vi "Test - Draw Teapot.vi"() -> ()   [LabVIEW 2022 SP3, in "Raster.lvlib"] (continued)
"y"=282.48926, "z"=0.9893855}, "UV"={"u"=0.0, "v"=0.0}, "Colour"=12517256}, "Vertex 2"={"Position"={"x"=187.54259, "y"=266.03958, "z"=0.9893693}, "UV"={"u"=0.0, "v"=0.0}, "Colour"=12517256}, "Vertex 3"={"Position"={"x"=198.46721, "y"=268.20078, "z"=0.990049}, "UV"={"u"=0.0, "v"=0.0}, "Colour"=12517256}, "Alpha"=0.0, "Alpha Blending Enabled"=FALSE, "Colour"=3162146}, {"Vertex 1"={"Position"={"x"=612.4574, "y"=266.03958, "z"=0.9893693}, "UV"={"u"=0.0, "v"=0.0}, "Colour"=12517256}, "Vertex 2"={"Position"={"x"=607.4049, "y"=282.48926, "z"=0.9893855}, "UV"={"u"=0.0, "v"=0.0}, "Colour"=12517256}, "Vertex 3"={"Position"={"x"=597.03815, "y"=283.57877, "z"=0.990049}, "UV"={"u"=0.0, "v"=0.0}, "Colour"=12517256}, "Alpha"=0.0, "Alpha Blending Enabled"=FALSE, "Colour"=3162146}, {"Vertex 1"={"Position"={"x"=430.5626, "y"=409.63797, "z"=0.98946077}, "UV"={"u"=0.0, "v"=0.0}, "Colour"=12517256}, "Vertex 2"={"Position"={"x"=421.46735, "y"=411.46152, "z"=0.9896358}, "UV"={"u"=0.0, "v"=0.0}, "Colour"=12517256}, "Vertex 3"={"Position"={"x"=424.30502, "y"=410.7137, "z"=0.9897057}, "UV"={"u"=0.0, "v"=0.0}, "Colour"=12517256}, "Alpha"=0.0, "Alpha Blending Enabled"=FALSE, "Colour"=10145390}, {"Vertex 1"={"Position"={"x"=385.91513, "y"=432.98935, "z"=0.9896798}, "UV"={"u"=0.0, "v"=0.0}, "Colour"=12517256}, "Vertex 2"={"Position"={"x"=382.30276, "y"=440.7109, "z"=0.9895852}, "UV"={"u"=0.0, "v"=0.0}, "Colour"=12517256}, "Vertex 3"={"Position"={"x"=386.13464, "y"=441.3613, "z"=0.9895369}, "UV"={"u"=0.0, "v"=0.0}, "Colour"=12517256}, "Alpha"=0.0, "Alpha Blending Enabled"=FALSE, "Colour"=131841}, {"Vertex 1"={"Position"={"x"=186.5184, "y"=191.99817, "z"=0.98936605}, "UV"={"u"=0.0, "v"=0.0}, "Colour"=12517256}, "Vertex 2"={"Position"={"x"=193.06175, "y"=180.83313, "z"=0.989387}, "UV"={"u"=0.0, "v"=0.0}, "Colour"=12517256}, "Vertex 3"={"Position"={"x"=203.37758, "y"=188.23193, "z"=0.990049}, "UV"={"u"=0.0, "v"=0.0}, "Colour"=12517256}, "Alpha"=0.0, "Alpha Blending Enabled"=FALSE, "Colour"=131841}, {"Vertex 1"={"Position"={"x"=606.9383, "y"=180.83313, "z"=0.989387}, "UV"={"u"=0.0, "v"=0.0}, "Colour"=12517256}, "Vertex 2"={"Position"={"x"=613.4816, "y"=191.99817, "z"=0.98936605}, "UV"={"u"=0.0, "v"=0.0}, "Colour"=12517256}, "Vertex 3"={"Position"={"x"=602.44214, "y"=198.90225, "z"=0.990049}, "UV"={"u"=0.0, "v"=0.0}, "Colour"=12517256}, "Alpha"=0.0, "Alpha Blending Enabled"=FALSE, "Colour"=131841}, {"Vertex 1"={"Position"={"x"=425.17258, "y"=447.3146, "z"=0.98956454}, "UV"={"u"=0.0, "v"=0.0}, "Colour"=12517256}, "Vertex 2"={"Position"={"x"=421.02798, "y"=439.917, "z"=0.9896443}, "UV"={"u"=0.0, "v"=0.0}, "Colour"=12517256}, "Vertex 3"={"Position"={"x"=417.69724, "y"=440.7109, "z"=0.9895852}, "UV"={"u"=0.0, "v"=0.0}, "Colour"=12517256}, "Alpha"=0.0, "Alpha Blending Enabled"=FALSE, "Colour"=131841}, {"Vertex 1"={"Position"={"x"=299.91116, "y"=121.74838, "z"=0.98940194}, "UV"={"u"=0.0, "v"=0.0}, "Colour"=12517256}, "Vertex 2"={"Position"={"x"=327.3322, "y"=123.64719, "z"=0.9895792}, "UV"={"u"=0.0, "v"=0.0}, "Colour"=12517256}, "Vertex 3"={"Position"={"x"=326.15854, "y"=127.58133, "z"=0.9898128}, "UV"={"u"=0.0, "v"=0.0}, "Colour"=12517256}, "Alpha"=0.0, "Alpha Blending Enabled"=FALSE, "Colour"=131841}, {"Vertex 1"={"Position"={"x"=413.86533, "y"=441.3613, "z"=0.9895369}, "UV"={"u"=0.0, "v"=0.0}, "Colour"=12517256}, "Vertex 2"={"Position"={"x"=411.0237, "y"=433.47845, "z"=0.9896417}, "UV"={"u"=0.0, "v"=0.0}, "Colour"=12517256}, "Vertex 3"={"Position"={"x"=407.6209, "y"=433.84442, "z"=0.9896132}, "UV"={"u"=0.0, "v"=0.0}, "Colour"=12517256}, "Alpha"=0.0, "Alpha Blending Enabled"=FALSE, "Colour"=131842}, {"Vertex 1"={"Position"={"x"=521.88995, "y"=127.45417, "z"=0.9896591}, "UV"={"u"=0.0, "v"=0.0}, "Colour"=12517256}, "Vertex 2"={"Position"={"x"=500.85635, "y"=127.179695, "z"=0.98972636}, "UV"={"u"=0.0, "v"=0.0}, "Colour"=12517256}, "Vertex 3"={"Position"={"x"=500.08884, "y"=121.74838, "z"=0.98940194}, "UV"={"u"=0.0, "v"=0.0}, "Colour"=12517256}, "Alpha"=0.0, "Alpha Blending Enabled"=FALSE, "Colour"=131841}, {"Vertex 1"={"Position"={"x"=677.0391, "y"=342.4919, "z"=0.9896034}, "UV"={"u"=0.0, "v"=0.0}, "Colour"=12517256}, "Vertex 2"={"Position"={"x"=673.70026, "y"=326.4925, "z"=0.98952615}, "UV"={"u"=0.0, "v"=0.0}, "Colour"=12517256}, "Vertex 3"={"Position"={"x"=666.5026, "y"=329.28787, "z"=0.9896555}, "UV"={"u"=0.0, "v"=0.0}, "Colour"=12517256}, "Alpha"=0.0, "Alpha Blending Enabled"=FALSE, "Colour"=8696158}, {"Vertex 1"={"Position"={"x"=282.90906, "y"=394.1647, "z"=0.98967445}, "UV"={"u"=0.0, "v"=0.0}, "Colour"=12517256}, "Vertex 2"={"Position"={"x"=297.17767, "y"=396.39102, "z"=0.98972005}, "UV"={"u"=0.0, "v"=0.0}, "Colour"=12517256}, "Vertex 3"={"Position"={"x"=297.89752, "y"=399.48126, "z"=0.9893889}, "UV"={"u"=0.0, "v"=0.0}, "Colour"=12517256}, "Alpha"=0.0, "Alpha Blending Enabled"=FALSE, "Colour"=9091427}, {"Vertex 1"={"Position"={"x"=426.9856, "y"=460.57834, "z"=0.9896675}, "UV"={"u"=0.0, "v"=0.0}, "Colour"=12517256}, "Vertex 2"={"Position"={"x"=431.49448, "y"=457.60767, "z"=0.98960376}, "UV"={"u"=0.0, "v"=0.0}, "Colour"=12517256}, "Vertex 3"={"Position"={"x"=427.8845, "y"=458.98697, "z"=0.9895123}, "UV"={"u"=0.0, "v"=0.0}, "Colour"=12517256}, "Alpha"=0.0, "Alpha Blending Enabled"=FALSE, "Colour"=10540914}, {"Vertex 1"={"Position"={"x"=390.02243, "y"=415.3864, "z"=0.9896799}, "UV"={"u"=0.0, "v"=0.0}, "Colour"=12517256}, "Vertex 2"={"Position"={"x"=385.85406, "y"=412.64026, "z"=0.98952574}, "UV"={"u"=0.0, "v"=0.0}, "Colour"=12517256}, "Vertex 3"={"Position"={"x"=381.9381, "y"=412.10922, "z"=0.98957527}, "UV"={"u"=0.0, "v"=0.0}, "Colour"=12517256}, "Alpha"=0.0, "Alpha Blending Enabled"=FALSE, "Colour"=11331451}, {"Vertex 1"={"Position"={"x"=410.90912, "y"=464.3185, "z"=0.98942566}, "UV"={"u"=0.0, "v"=0.0}, "Colour"=12517256}, "Vertex 2"={"Position"={"x"=406.71997, "y"=463.19003, "z"=0.98966503}, "UV"={"u"=0.0, "v"=0.0}, "Colour"=12517256}, "Vertex 3"={"Position"={"x"=409.72174, "y"=462.79736, "z"=0.98969}, "UV"={"u"=0.0, "v"=0.0}, "Colour"=12517256}, "Alpha"=0.0, "Alpha Blending Enabled"=FALSE, "Colour"=10343280}, {"Vertex 1"={"Position"={"x"=390.2171, "y"=413.03857, "z"=0.9894885}, "UV"={"u"=0.0, "v"=0.0}, "Colour"=12517256}, "Vertex 2"={"Position"={"x"=393.107, "y"=415.6739, "z"=0.98965406}, "UV"={"u"=0.0, "v"=0.0}, "Colour"=12517256}, "Vertex 3"={"Position"={"x"=396.44946, "y"=415.85388, "z"=0.98963785}, "UV"={"u"=0.0, "v"=0.0}, "Colour"=12517256}, "Alpha"=0.0, "Alpha Blending Enabled"=FALSE, "Colour"=11792768}, {"Vertex 1"={"Position"={"x"=648.53705, "y"=216.88268, "z"=0.98970413}, "UV"={"u"=0.0, "v"=0.0}, "Colour"=12517256}, "Vertex 2"={"Position"={"x"=621.5498, "y"=201.64421, "z"=0.9896861}, "UV"={"u"=0.0, "v"=0.0}, "Colour"=12517256}, "Vertex 3"={"Position"={"x"=626.93384, "y"=205.09799, "z"=0.989385}, "UV"={"u"=0.0, "v"=0.0}, "Colour"=12517256}, "Alpha"=0.0, "Alpha Blending Enabled"=FALSE, "Colour"=131841}, {"Vertex 1"={"Position"={"x"=187.54259, "y"=266.03958, "z"=0.9893693}, "UV"={"u"=0.0, "v"=0.0}, "Colour"=12517256}, "Vertex 2"={"Position"={"x"=183.7062, "y"=249.90852, "z"=0.98935705}, "UV"={"u"=0.0, "v"=0.0}, "Colour"=12517256}, "Vertex 3"={"Position"={"x"=195.06374, "y"=253.1501, "z"=0.990049}, "UV"={"u"=0.0, "v"=0.0}, "Colour"=12517256}, "Alpha"=0.0, "Alpha Blending Enabled"=FALSE, "Colour"=2635036}, {"Vertex 1"={"Position"={"x"=616.2938, "y"=249.90852, "z"=0.98935705}, "UV"={"u"=0.0, "v"=0.0}, "Colour"=12517256}, "Vertex 2"={"Position"={"x"=612.4574, "y"=266.03958, "z"=0.9893693}, "UV"={"u"=0.0, "v"=0.0}, "Colour"=12517256}, "Vertex 3"={"Position"={"x"=601.5328, "y"=268.20078, "z"=0.990049}, "UV"={"u"=0.0, "v"=0.0}, "Colour"=12517256}, "Alpha"=0.0, "Alpha Blending Enabled"=FALSE, "Colour"=2635036}, {"Vertex 1"={"Position"={"x"=662.8395, "y"=314.53314, "z"=0.9895922}, "UV"={"u"=0.0, "v"=0.0}, "Colour"=12517256}, "Vertex 2"={"Position"={"x"=666.5026, "y"=329.28787, "z"=0.9896555}, "UV"={"u"=0.0, "v"=0.0}, "Colour"=12517256}, "Vertex 3"={"Position"={"x"=673.70026, "y"=326.4925, "z"=0.98952615}, "UV"={"u"=0.0, "v"=0.0}, "Colour"=12517256}, "Alpha"=0.0, "Alpha Blending Enabled"=FALSE, "Colour"=8696158}, {"Vertex 1"={"Position"={"x"=189.80782, "y"=199.68152, "z"=0.98959744}, "UV"={"u"=0.0, "v"=0.0}, "Colour"=12517256}, "Vertex 2"={"Position"={"x"=169.41815, "y"=209.785, "z"=0.98959744}, "UV"={"u"=0.0, "v"=0.0}, "Colour"=12517256}, "Vertex 3"={"Position"={"x"=168.53177, "y"=213.96883, "z"=0.9895778}, "UV"={"u"=0.0, "v"=0.0}, "Colour"=12517256}, "Alpha"=0.0, "Alpha Blending Enabled"=FALSE, "Colour"=6522183}, {"Vertex 1"={"Position"={"x"=168.51642, "y"=218.47636, "z"=0.98959744}, "UV"={"u"=0.0, "v"=0.0}, "Colour"=12517256}, "Vertex 2"={"Position"={"x"=186.59279, "y"=209.32652, "z"=0.98959744}, "UV"={"u"=0.0, "v"=0.0}, "Colour"=12517256}, "Vertex 3"={"Position"={"x"=187.80107, "y"=204.32404, "z"=0.9895778}, "UV"={"u"=0.0, "v"=0.0}, "Colour"=12517256}, "Alpha"=0.0, "Alpha Blending Enabled"=FALSE, "Colour"=10606707}, {"Vertex 1"={"Position"={"x"=169.41815, "y"=209.785, "z"=0.98959744}, "UV"={"u"=0.0, "v"=0.0}, "Colour"=12517256}, "Vertex 2"={"Position"={"x"=151.36185, "y"=220.60233, "z"=0.98959744}, "UV"={"u"=0.0, "v"=0.0}, "Colour"=12517256}, "Vertex 3"={"Position"={"x"=151.49875, "y"=224.43393, "z"=0.9895778}, "UV"={"u"=0.0, "v"=0.0}, "Colour"=12517256}, "Alpha"=0.0, "Alpha Blending Enabled"=FALSE, "Colour"=6653768}, {"Vertex 1"={"Position"={"x"=152.57072, "y"=228.54994, "z"=0.98959744}, "UV"={"u"=0.0, "v"=0.0}, "Colour"=12517256}, "Vertex 2"={"Position"={"x"=168.51642, "y"=218.47636, "z"=0.98959744}, "UV"={"u"=0.0, "v"=0.0}, "Colour"=12517256}, "Vertex 3"={"Position"={"x"=168.53177, "y"=213.96883, "z"=0.9895778}, "UV"={"u"=0.0, "v"=0.0}, "Colour"=12517256}, "Alpha"=0.0, "Alpha Blending Enabled"=FALSE, "Colour"=10540915}, {"Vertex 1"={"Position"={"x"=151.36185, "y"=220.60233, "z"=0.98959744}, "UV"={"u"=0.0, "v"=0.0}, "Colour"=12517256}, "Vertex 2"={"Position"={"x"=135.59482, "y"=232.01439, "z"=0.98959744}, "UV"={"u"=0.0, "v"=0.0}, "Colour"=12517256}, "Vertex 3"={"Position"={"x"=136.65297, "y"=235.5601, "z"=0.9895778}, "UV"={"u"=0.0, "v"=0.0}, "Colour"=12517256}, "Alpha"=0.0, "Alpha Blending Enabled"=FALSE, "Colour"=6851402}, {"Vertex 1"={"Position"={"x"=138.70209, "y"=239.3482, "z"=0.98959744}, "UV"={"u"=0.0, "v"=0.0}, "Colour"=12517256}, "Vertex 2"={"Position"={"x"=152.57072, "y"=228.54994, "z"=0.98959744}, "UV"={"u"=0.0, "v"=0.0}, "Colour"=12517256}, "Vertex 3"={"Position"={"x"=151.49875, "y"=224.43393, "z"=0.9895778}, "UV"={"u"=0.0, "v"=0.0}, "Colour"=12517256}, "Alpha"=0.0, "Alpha Blending Enabled"=FALSE, "Colour"=10409073}, {"Vertex 1"={"Position"={"x"=135.59482, "y"=232.01439, "z"=0.98959744}, "UV"={"u"=0.0, "v"=0.0}, "Colour"=12517256}, "Vertex 2"={"Position"={"x"=122.07298, "y"=243.90215, "z"=0.98959744}, "UV"={"u"=0.0, "v"=0.0}, "Colour"=12517256}, "Vertex 3"={"Position"={"x"=123.94555, "y"=247.18822, "z"=0.9895778}, "UV"={"u"=0.0, "v"=0.0}, "Colour"=12517256}, "Alpha"=0.0, "Alpha Blending Enabled"=FALSE, "Colour"=7049293}, {"Vertex 1"={"Position"={"x"=126.85683, "y"=250.67299, "z"=0.98959744}, "UV"={"u"=0.0, "v"=0.0}, "Colour"=12517256}, "Vertex 2"={"Position"={"x"=138.70209, "y"=239.3482, "z"=0.98959744}, "UV"={"u"=0.0, "v"=0.0}, "Colour"=12517256}, "Vertex 3"={"Position"={"x"=136.65297, "y"=235.5601, "z"=0.9895778}, "UV"={"u"=0.0, "v"=0.0}, "Colour"=12517256}, "Alpha"=0.0, "Alpha Blending Enabled"=FALSE, "Colour"=10211183}, {"Vertex 1"={"Position"={"x"=122.07298, "y"=243.90215, "z"=0.98959744}, "UV"={"u"=0.0, "v"=0.0}, "Colour"=12517256}, "Vertex 2"={"Position"={"x"=110.75225, "y"=256.14658, "z"=0.98959744}, "UV"={"u"=0.0, "v"=0.0}, "Colour"=12517256}, "Vertex 3"={"Position"={"x"=113.32741, "y"=259.15903, "z"=0.9895778}, "UV"={"u"=0.0, "v"=0.0}, "Colour"=12517256}, "Alpha"=0.0, "Alpha Blending Enabled"=FALSE, "Colour"=7312720}, {"Vertex 1"={"Position"={"x"=116.981316, "y"=262.32532, "z"=0.98959744}, "UV"={"u"=0.0, "v"=0.0}, "Colour"=12517256}, "Vertex 2"={"Position"={"x"=126.85683, "y"=250.67299, "z"=0.98959744}, "UV"={"u"=0.0, "v"=0.0}, "Colour"=12517256}, "Vertex 3"={"Position"={"x"=123.94555, "y"=247.18822, "z"=0.9895778}, "UV"={"u"=0.0, "v"=0.0}, "Colour"=12517256}, "Alpha"=0.0, "Alpha Blending Enabled"=FALSE, "Colour"=9948012}, {"Vertex 1"={"Position"={"x"=110.75225, "y"=256.14658, "z"=0.98959744}, "UV"={"u"=0.0, "v"=0.0}, "Colour"=12517256}, "Vertex 2"={"Position"={"x"=101.588585, "y"=268.6284, "z"=0.98959744}, "UV"={"u"=0.0, "v"=0.0}, "Colour"=12517256}, "Vertex 3"={"Position"={"x"=104.74968, "y"=271.31357, "z"=0.9895778}, "UV"={"u"=0.0, "v"=0.0}, "Colour"=12517256}, "Alpha"=0.0, "Alpha Blending Enabled"=FALSE, "Colour"=7576146}, {"Vertex 1"={"Position"={"x"=109.02176, "y"=274.10672, "z"=0.98959744}, "UV"={"u"=0.0, "v"=0.0}, "Colour"=12517256}, "Vertex 2"={"Position"={"x"=116.981316, "y"=262.32532, "z"=0.98959744}, "UV"={"u"=0.0, "v"=0.0}, "Colour"=12517256}, "Vertex 3"={"Position"={"x"=113.32741, "y"=259.15903, "z"=0.9895778}, "UV"={"u"=0.0, "v"=0.0}, "Colour"=12517256}, "Alpha"=0.0, "Alpha Blending Enabled"=FALSE, "Colour"=9750122}, {"Vertex 1"={"Position"={"x"=101.588585, "y"=268.6284, "z"=0.98959744}, "UV"={"u"=0.0, "v"=0.0}, "Colour"=12517256}, "Vertex 2"={"Position"={"x"=94.53805, "y"=281.22873, "z"=0.98959744}, "UV"={"u"=0.0, "v"=0.0}, "Colour"=12517256}, "Vertex 3"={"Position"={"x"=98.163345, "y"=283.49265, "z"=0.9895778}, "UV"={"u"=0.0, "v"=0.0}, "Colour"=12517256}, "Alpha"=0.0, "Alpha Blending Enabled"=FALSE, "Colour"=7774037}, {"Vertex 1"={"Position"={"x"=102.92444, "y"=285.8186, "z"=0.98959744}, "UV"={"u"=0.0, "v"=0.0}, "Colour"=12517256}, "Vertex 2"={"Position"={"x"=109.02176, "y"=274.10672, "z"=0.98959744}, "UV"={"u"=0.0, "v"=0.0}, "Colour"=12517256}, "Vertex 3"={"Position"={"x"=104.74968, "y"=271.31357, "z"=0.9895778}, "UV"={"u"=0.0, "v"=0.0}, "Colour"=12517256}, "Alpha"=0.0, "Alpha Blending Enabled"=FALSE, "Colour"=9486951}, {"Vertex 1"={"Position"={"x"=94.53805, "y"=281.22873, "z"=0.98959744}, "UV"={"u"=0.0, "v"=0.0}, "Colour"=12517256}, "Vertex 2"={"Position"={"x"=89.5565, "y"=293.82855, "z"=0.98959744}, "UV"={"u"=0.0, "v"=0.0}, "Colour"=12517256}, "Vertex 3"={"Position"={"x"=93.51947, "y"=295.5369, "z"=0.9895778}, "UV"={"u"=0.0, "v"=0.0}, "Colour"=12517256}, "Alpha"=0.0, "Alpha Blending Enabled"=FALSE, "Colour"=8037463}, {"Vertex 1"={"Position"={"x"=98.63565, "y"=297.2621, "z"=0.98959744}, "UV"={"u"=0.0, "v"=0.0}, "Colour"=12517256}, "Vertex 2"={"Position"={"x"=102.92444, "y"=285.8186, "z"=0.98959744}, "UV"={"u"=0.0, "v"=0.0}, "Colour"=12517256}, "Vertex 3"={"Position"={"x"=98.163345, "y"=283.49265, "z"=0.9895778}, "UV"={"u"=0.0, "v"=0.0}, "Colour"=12517256}, "Alpha"=0.0, "Alpha Blending Enabled"=FALSE, "Colour"=9289061}, {"Vertex 1"={"Position"={"x"=89.5565, "y"=293.82855, "z"=0.98959744}, "UV"={"u"=0.0, "v"=0.0}, "Colour"=12517256}, "Vertex 2"={"Position"={"x"=86.5999, "y"=306.30865, "z"=0.98959744}, "UV"={"u"=0.0, "v"=0.0}, "Colour"=12517256}, "Vertex 3"={"Position"={"x"=90.76903, "y"=307.28738, "z"=0.9895778}, "UV"={"u"=0.0, "v"=0.0}, "Colour"=12517256}, "Alpha"=0.0, "Alpha Blending Enabled"=FALSE, "Colour"=8300890}, {"Vertex 1"={"Position"={"x"=96.10178, "y"=308.23883, "z"=0.98959744}, "UV"={"u"=0.0, "v"=0.0}, "Colour"=12517256}, "Vertex 2"={"Position"={"x"=98.63565, "y"=297.2621, "z"=0.98959744}, "UV"={"u"=0.0, "v"=0.0}, "Colour"=12517256}, "Vertex 3"={"Position"={"x"=93.51947, "y"=295.5369, "z"=0.9895778}, "UV"={"u"=0.0, "v"=0.0}, "Colour"=12517256}, "Alpha"=0.0, "Alpha Blending Enabled"=FALSE, "Colour"=9091427}, {"Vertex 1"={"Position"={"x"=86.5999, "y"=306.30865, "z"=0.98959744}, "UV"={"u"=0.0, "v"=0.0}, "Colour"=12517256}, "Vertex 2"={"Position"={"x"=85.62412, "y"=318.55002, "z"=0.98959744}, "UV"={"u"=0.0, "v"=0.0}, "Colour"=12517256}, "Vertex 3"={"Position"={"x"=89.86314, "y"=318.58496, "z"=0.9895778}, "UV"={"u"=0.0, "v"=0.0}, "Colour"=12517256}, "Alpha"=0.0, "Alpha Blending Enabled"=FALSE, "Colour"=8564317}, {"Vertex 1"={"Position"={"x"=95.26916, "y"=318.55002, "z"=0.98959744}, "UV"={"u"=0.0, "v"=0.0}, "Colour"=12517256}, "Vertex 2"={"Position"={"x"=96.10178, "y"=308.23883, "z"=0.98959744}, "UV"={"u"=0.0, "v"=0.0}, "Colour"=12517256}, "Vertex 3"={"Position"={"x"=90.76903, "y"=307.28738, "z"=0.9895778}, "UV"={"u"=0.0, "v"=0.0}, "Colour"=12517256}, "Alpha"=0.0, "Alpha Blending Enabled"=FALSE, "Colour"=8828000}, {"Vertex 1"={"Position"={"x"=85.62412, "y"=318.55002, "z"=0.98959744}, "UV"={"u"=0.0, "v"=0.0}, "Colour"=12517256}, "Vertex 2"={"Position"={"x"=87.13484, "y"=329.46445, "z"=0.98959744}, "UV"={"u"=0.0, "v"=0.0}, "Colour"=12517256}, "Vertex 3"={"Position"={"x"=91.32674, "y"=328.538, "z"=0.9895778}, "UV"={"u"=0.0, "v"=0.0}, "Colour"=12517256}, "Alpha"=0.0, "Alpha Blending Enabled"=FALSE, "Colour"=8894049}, {"Vertex 1"={"Position"={"x"=96.68016, "y"=327.50403, "z"=0.98959744}, "UV"={"u"=0.0, "v"=0.0}, "Colour"=12517256}, "Vertex 2"={"Position"={"x"=95.26916, "y"=318.55002, "z"=0.98959744}, "UV"={"u"=0.0, "v"=0.0}, "Colour"=12517256}, "Vertex 3"={"Position"={"x"=89.86314, "y"=318.58496, "z"=0.9895778}, "UV"={"u"=0.0, "v"=0.0}, "Colour"=12517256}, "Alpha"=0.0, "Alpha Blending Enabled"=FALSE, "Colour"=8366939}, {"Vertex 1"={"Position"={"x"=87.13484, "y"=329.46445, "z"=0.98959744}, "UV"={"u"=0.0, "v"=0.0}, "Colour"=12517256}, "Vertex 2"={"Position"={"x"=91.65158, "y"=338.20395, "z"=0.98959744}, "UV"={"u"=0.0, "v"=0.0}, "Colour"=12517256}, "Vertex 3"={"Position"={"x"=95.695854, "y"=336.50763, "z"=0.9895778}, "UV"={"u"=0.0, "v"=0.0}, "Colour"=12517256}, "Alpha"=0.0, "Alpha Blending Enabled"=FALSE, "Colour"=9486695}, {"Vertex 1"={"Position"={"x"=100.88518, "y"=334.67392, "z"=0.98959744}, "UV"={"u"=0.0, "v"=0.0}, "Colour"=12517256}, "Vertex 2"={"Position"={"x"=96.68016, "y"=327.50403, "z"=0.98959744}, "UV"={"u"=0.0, "v"=0.0}, "Colour"=12517256}, "Vertex 3"={"Position"={"x"=91.32674, "y"=328.538, "z"=0.9895778}, "UV"={"u"=0.0, "v"=0.0}, "Colour"=12517256}, "Alpha"=0.0, "Alpha Blending Enabled"=FALSE, "Colour"=7707988}, {"Vertex 1"={"Position"={"x"=91.65158, "y"=338.20395, "z"=0.98959744}, "UV"={"u"=0.0, "v"=0.0}, "Colour"=12517256}, "Vertex 2"={"Position"={"x"=99.15168, "y"=345.0104, "z"=0.98959744}, "UV"={"u"=0.0, "v"=0.0}, "Colour"=12517256}, "Vertex 3"={"Position"={"x"=102.93782, "y"=342.71442, "z"=0.9895778}, "UV"={"u"=0.0, "v"=0.0}, "Colour"=12517256}, "Alpha"=0.0, "Alpha Blending Enabled"=FALSE, "Colour"=10013805}, {"Vertex 1"={"Position"={"x"=107.84178, "y"=340.25775, "z"=0.98959744}, "UV"={"u"=0.0, "v"=0.0}, "Colour"=12517256}, "Vertex 2"={"Position"={"x"=100.88518, "y"=334.67392, "z"=0.98959744}, "UV"={"u"=0.0, "v"=0.0}, "Colour"=12517256}, "Vertex 3"={"Position"={"x"=95.695854, "y"=336.50763, "z"=0.9895778}, "UV"={"u"=0.0, "v"=0.0}, "Colour"=12517256}, "Alpha"=0.0, "Alpha Blending Enabled"=FALSE, "Colour"=7114829}, {"Vertex 1"={"Position"={"x"=99.15168, "y"=345.0104, "z"=0.98959744}, "UV"={"u"=0.0, "v"=0.0}, "Colour"=12517256}, "Vertex 2"={"Position"={"x"=109.61189, "y"=350.12524, "z"=0.98959744}, "UV"={"u"=0.0, "v"=0.0}, "Colour"=12517256}, "Vertex 3"={"Position"={"x"=113.01999, "y"=347.37875, "z"=0.9895778}, "UV"={"u"=0.0, "v"=0.0}, "Colour"=12517256}, "Alpha"=0.0, "Alpha Blending Enabled"=FALSE, "Colour"=10409073}, {"Vertex 1"={"Position"={"x"=117.50798, "y"=344.45398, "z"=0.98959744}, "UV"={"u"=0.0, "v"=0.0}, "Colour"=12517256}, "Vertex 2"={"Position"={"x"=107.84178, "y"=340.25775, "z"=0.98959744}, "UV"={"u"=0.0, "v"=0.0}, "Colour"=12517256}, "Vertex 3"={"Position"={"x"=102.93782, "y"=342.71442, "z"=0.9895778}, "UV"={"u"=0.0, "v"=0.0}, "Colour"=12517256}, "Alpha"=0.0, "Alpha Blending Enabled"=FALSE, "Colour"=6588232}, {"Vertex 1"={"Position"={"x"=109.61189, "y"=350.12524, "z"=0.98959744}, "UV"={"u"=0.0, "v"=0.0}, "Colour"=12517256}, "Vertex 2"={"Position"={"x"=123.00947, "y"=353.7902, "z"=0.98959744}, "UV"={"u"=0.0, "v"=0.0}, "Colour"=12517256}, "Vertex 3"={"Position"={"x"=125.90974, "y"=350.72086, "z"=0.9895778}, "UV"={"u"=0.0, "v"=0.0}, "Colour"=12517256}, "Alpha"=0.0, "Alpha Blending Enabled"=FALSE, "Colour"=10672500}, {"Vertex 1"={"Position"={"x"=129.84137, "y"=347.46066, "z"=0.98959744}, "UV"={"u"=0.0, "v"=0.0}, "Colour"=12517256}, "Vertex 2"={"Position"={"x"=117.50798, "y"=344.45398, "z"=0.98959744}, "UV"={"u"=0.0, "v"=0.0}, "Colour"=12517256}, "Vertex 3"={"Position"={"x"=113.01999, "y"=347.37875, "z"=0.9895778}, "UV"={"u"=0.0, "v"=0.0}, "Colour"=12517256}, "Alpha"=0.0, "Alpha Blending Enabled"=FALSE, "Colour"=6324549}, {"Vertex 1"={"Position"={"x"=123.00947, "y"=353.7902, "z"=0.98959744}, "UV"={"u"=0.0, "v"=0.0}, "Colour"=12517256}, "Vertex 2"={"Position"={"x"=139.3214, "y"=356.247, "z"=0.98959744}, "UV"={"u"=0.0, "v"=0.0}, "Colour"=12517256}, "Vertex 3"={"Position"={"x"=141.57439, "y"=352.9612, "z"=0.9895778}, "UV"={"u"=0.0, "v"=0.0}, "Colour"=12517256}, "Alpha"=0.0, "Alpha Blending Enabled"=FALSE, "Colour"=10738549}, {"Vertex 1"={"Position"={"x"=144.79973, "y"=349.47617, "z"=0.98959744}, "UV"={"u"=0.0, "v"=0.0}, "Colour"=12517256}, "Vertex 2"={"Position"={"x"=129.84137, "y"=347.46066, "z"=0.98959744}, "UV"={"u"=0.0, "v"=0.0}, "Colour"=12517256}, "Vertex 3"={"Position"={"x"=125.90974, "y"=350.72086, "z"=0.9895778}, "UV"={"u"=0.0, "v"=0.0}, "Colour"=12517256}, "Alpha"=0.0, "Alpha Blending Enabled"=FALSE, "Colour"=6258500}, {"Vertex 1"={"Position"={"x"=139.3214, "y"=356.247, "z"=0.98959744}, "UV"={"u"=0.0, "v"=0.0}, "Colour"=12517256}, "Vertex 2"={"Position"={"x"=158.52467, "y"=357.73706, "z"=0.98959744}, "UV"={"u"=0.0, "v"=0.0}, "Colour"=12517256}, "Vertex 3"={"Position"={"x"=159.98125, "y"=354.3201, "z"=0.9895778}, "UV"={"u"=0.0, "v"=0.0}, "Colour"=12517256}, "Alpha"=0.0, "Alpha Blending Enabled"=FALSE, "Colour"=10804598}, {"Vertex 1"={"Position"={"x"=162.341, "y"=350.69873, "z"=0.98959744}, "UV"={"u"=0.0, "v"=0.0}, "Colour"=12517256}, "Vertex 2"={"Position"={"x"=144.79973, "y"=349.47617, "z"=0.98959744}, "UV"={"u"=0.0, "v"=0.0}, "Colour"=12517256}, "Vertex 3"={"Position"={"x"=141.57439, "y"=352.9612, "z"=0.9895778}, "UV"={"u"=0.0, "v"=0.0}, "Colour"=12517256}, "Alpha"=0.0, "Alpha Blending Enabled"=FALSE, "Colour"=6192707}, {"Vertex 1"={"Position"={"x"=158.52467, "y"=357.73706, "z"=0.98959744}, "UV"={"u"=0.0, "v"=0.0}, "Colour"=12517256}, "Vertex 2"={"Position"={"x"=180.59659, "y"=358.50238, "z"=0.98959744}, "UV"={"u"=0.0, "v"=0.0}, "Colour"=12517256}, "Vertex 3"={"Position"={"x"=181.09776, "y"=355.0179, "z"=0.9895778}, "UV"={"u"=0.0, "v"=0.0}, "Colour"=12517256}, "Alpha"=0.0, "Alpha Blending Enabled"=FALSE, "Colour"=10870134}, {"Vertex 1"={"Position"={"x"=182.42264, "y"=351.32635, "z"=0.98959744}, "UV"={"u"=0.0, "v"=0.0}, "Colour"=12517256}, "Vertex 2"={"Position"={"x"=162.341, "y"=350.69873, "z"=0.98959744}, "UV"={"u"=0.0, "v"=0.0}, "Colour"=12517256}, "Vertex 3"={"Position"={"x"=159.98125, "y"=354.3201, "z"=0.9895778}, "UV"={"u"=0.0, "v"=0.0}, "Colour"=12517256}, "Alpha"=0.0, "Alpha Blending Enabled"=FALSE, "Colour"=6192707}, {"Vertex 1"={"Position"={"x"=180.59659, "y"=358.50238, "z"=0.98959744}, "UV"={"u"=0.0, "v"=0.0}, "Colour"=12517256}, "Vertex 2"={"Position"={"x"=205.5139, "y"=358.7842, "z"=0.98959744}, "UV"={"u"=0.0, "v"=0.0}, "Colour"=12517256}, "Vertex 3"={"Position"={"x"=204.89125, "y"=355.27502, "z"=0.9895778}, "UV"={"u"=0.0, "v"=0.0}, "Colour"=12517256}, "Alpha"=0.0, "Alpha Blending Enabled"=FALSE, "Colour"=10870134}, {"Vertex 1"={"Position"={"x"=205.00276, "y"=351.5577, "z"=0.98959744}, "UV"={"u"=0.0, "v"=0.0}, "Colour"=12517256}, "Vertex 2"={"Position"={"x"=182.42264, "y"=351.32635, "z"=0.98959744}, "UV"={"u"=0.0, "v"=0.0}, "Colour"=12517256}, "Vertex 3"={"Position"={"x"=181.09776, "y"=355.0179, "z"=0.9895778}, "UV"={"u"=0.0, "v"=0.0}, "Colour"=12517256}, "Alpha"=0.0, "Alpha Blending Enabled"=FALSE, "Colour"=6192964}, {"Vertex 1"={"Position"={"x"=205.5139, "y"=358.7842, "z"=0.98959744}, "UV"={"u"=0.0, "v"=0.0}, "Colour"=12517256}, "Vertex 2"={"Position"={"x"=233.2539, "y"=358.82452, "z"=0.98959744}, "UV"={"u"=0.0, "v"=0.0}, "Colour"=12517256}, "Vertex 3"={"Position"={"x"=231.32906, "y"=355.31174, "z"=0.9895778}, "UV"={"u"=0.0, "v"=0.0}, "Colour"=12517256}, "Alpha"=0.0, "Alpha Blending Enabled"=FALSE, "Colour"=10870134}, {"Vertex 1"={"Position"={"x"=230.03891, "y"=351.59073, "z"=0.98959744}, "UV"={"u"=0.0, "v"=0.0}, "Colour"=12517256}, "Vertex 2"={"Position"={"x"=205.00276, "y"=351.5577, "z"=0.98959744}, "UV"={"u"=0.0, "v"=0.0}, "Colour"=12517256}, "Vertex 3"={"Position"={"x"=204.89125, "y"=355.27502, "z"=0.9895778}, "UV"={"u"=0.0, "v"=0.0}, "Colour"=12517256}, "Alpha"=0.0, "Alpha Blending Enabled"=FALSE, "Colour"=6258500}, {"Vertex 1"={"Position"={"x"=348.88834, "y"=405.76608, "z"=0.98953724}, "UV"={"u"=0.0, "v"=0.0}, "Colour"=12517256}, "Vertex 2"={"Position"={"x"=362.46423, "y"=407.4392, "z"=0.98967314}, "UV"={"u"=0.0, "v"=0.0}, "Colour"=12517256}, "Vertex 3"={"Position"={"x"=365.49564, "y"=408.5937, "z"=0.9895617}, "UV"={"u"=0.0, "v"=0.0}, "Colour"=12517256}, "Alpha"=0.0, "Alpha Blending Enabled"=FALSE, "Colour"=9618536}, {"Vertex 1"={"Position"={"x"=427.8845, "y"=458.98697, "z"=0.9895123}, "UV"={"u"=0.0, "v"=0.0}, "Colour"=12517256}, "Vertex 2"={"Position"={"x"=423.8626, "y"=461.78098, "z"=0.98958975}, "UV"={"u"=0.0, "v"=0.0}, "Colour"=12517256}, "Vertex 3"={"Position"={"x"=426.9856, "y"=460.57834, "z"=0.9896675}, "UV"={"u"=0.0, "v"=0.0}, "Colour"=12517256}, "Alpha"=0.0, "Alpha Blending Enabled"=FALSE, "Colour"=10540914}, {"Vertex 1"={"Position"={"x"=182.0637, "y"=204.669, "z"=0.98935175}, "UV"={"u"=0.0, "v"=0.0}, "Colour"=12517256}, "Vertex 2"={"Position"={"x"=186.5184, "y"=191.99817, "z"=0.98936605}, "UV"={"u"=0.0, "v"=0.0}, "Colour"=12517256}, "Vertex 3"={"Position"={"x"=197.55788, "y"=198.90225, "z"=0.990049}, "UV"={"u"=0.0, "v"=0.0}, "Colour"=12517256}, "Alpha"=0.0, "Alpha Blending Enabled"=FALSE, "Colour"=131841}, {"Vertex 1"={"Position"={"x"=613.4816, "y"=191.99817, "z"=0.98936605}, "UV"={"u"=0.0, "v"=0.0}, "Colour"=12517256}, "Vertex 2"={"Position"={"x"=617.93634, "y"=204.669, "z"=0.98935175}, "UV"={"u"=0.0, "v"=0.0}, "Colour"=12517256}, "Vertex 3"={"Position"={"x"=606.3912, "y"=210.88196, "z"=0.990049}, "UV"={"u"=0.0, "v"=0.0}, "Colour"=12517256}, "Alpha"=0.0, "Alpha Blending Enabled"=FALSE, "Colour"=131841}, {"Vertex 1"={"Position"={"x"=411.0237, "y"=433.47845, "z"=0.9896417}, "UV"={"u"=0.0, "v"=0.0}, "Colour"=12517256}, "Vertex 2"={"Position"={"x"=413.86533, "y"=441.3613, "z"=0.9895369}, "UV"={"u"=0.0, "v"=0.0}, "Colour"=12517256}, "Vertex 3"={"Position"={"x"=417.69724, "y"=440.7109, "z"=0.9895852}, "UV"={"u"=0.0, "v"=0.0}, "Colour"=12517256}, "Alpha"=0.0, "Alpha Blending Enabled"=FALSE, "Colour"=131841}, {"Vertex 1"={"Position"={"x"=371.54373, "y"=446.1597, "z"=0.9896467}, "UV"={"u"=0.0, "v"=0.0}, "Colour"=12517256}, "Vertex 2"={"Position"={"x"=368.48776, "y"=452.57986, "z"=0.9896035}, "UV"={"u"=0.0, "v"=0.0}, "Colour"=12517256}, "Vertex 3"={"Position"={"x"=372.0999, "y"=453.91602, "z"=0.98951197}, "UV"={"u"=0.0, "v"=0.0}, "Colour"=12517256}, "Alpha"=0.0, "Alpha Blending Enabled"=FALSE, "Colour"=197634}, {"Vertex 1"={"Position"={"x"=671.18396, "y"=239.12437, "z"=0.9894685}, "UV"={"u"=0.0, "v"=0.0}, "Colour"=12517256}, "Vertex 2"={"Position"={"x"=682.01483, "y"=260.7837, "z"=0.9895282}, "UV"={"u"=0.0, "v"=0.0}, "Colour"=12517256}, "Vertex 3"={"Position"={"x"=678.03265, "y"=257.92834, "z"=0.98976254}, "UV"={"u"=0.0, "v"=0.0}, "Colour"=12517256}, "Alpha"=0.0, "Alpha Blending Enabled"=FALSE, "Colour"=131841}, {"Vertex 1"={"Position"={"x"=405.04242, "y"=413.28833, "z"=0.9894651}, "UV"={"u"=0.0, "v"=0.0}, "Colour"=12517256}, "Vertex 2"={"Position"={"x"=403.55054, "y"=415.85388, "z"=0.98963785}, "UV"={"u"=0.0, "v"=0.0}, "Colour"=12517256}, "Vertex 3"={"Position"={"x"=406.89297, "y"=415.6739, "z"=0.98965406}, "UV"={"u"=0.0, "v"=0.0}, "Colour"=12517256}, "Alpha"=0.0, "Alpha Blending Enabled"=FALSE, "Colour"=11792768}, {"Vertex 1"={"Position"={"x"=390.40692, "y"=441.8486, "z"=0.98950064}, "UV"={"u"=0.0, "v"=0.0}, "Colour"=12517256}, "Vertex 2"={"Position"={"x"=392.3791, "y"=433.84442, "z"=0.9896132}, "UV"={"u"=0.0, "v"=0.0}, "Colour"=12517256}, "Vertex 3"={"Position"={"x"=388.97626, "y"=433.47845, "z"=0.9896417}, "UV"={"u"=0.0, "v"=0.0}, "Colour"=12517256}, "Alpha"=0.0, "Alpha Blending Enabled"=FALSE, "Colour"=131842}, {"Vertex 1"={"Position"={"x"=183.7062, "y"=249.90852, "z"=0.98935705}, "UV"={"u"=0.0, "v"=0.0}, "Colour"=12517256}, "Vertex 2"={"Position"={"x"=181.27118, "y"=234.16856, "z"=0.98934925}, "UV"={"u"=0.0, "v"=0.0}, "Colour"=12517256}, "Vertex 3"={"Position"={"x"=192.90733, "y"=238.47354, "z"=0.990049}, "UV"={"u"=0.0, "v"=0.0}, "Colour"=12517256}, "Alpha"=0.0, "Alpha Blending Enabled"=FALSE, "Colour"=1976341}, {"Vertex 1"={"Position"={"x"=618.7288, "y"=234.16856, "z"=0.98934925}, "UV"={"u"=0.0, "v"=0.0}, "Colour"=12517256}, "Vertex 2"={"Position"={"x"=616.2938, "y"=249.90852, "z"=0.98935705}, "UV"={"u"=0.0, "v"=0.0}, "Colour"=12517256}, "Vertex 3"={"Position"={"x"=604.9363, "y"=253.1501, "z"=0.990049}, "UV"={"u"=0.0, "v"=0.0}, "Colour"=12517256}, "Alpha"=0.0, "Alpha Blending Enabled"=FALSE, "Colour"=1976341}, {"Vertex 1"={"Position"={"x"=168.53177, "y"=213.96883, "z"=0.9895778}, "UV"={"u"=0.0, "v"=0.0}, "Colour"=12517256}, "Vertex 2"={"Position"={"x"=187.80107, "y"=204.32404, "z"=0.9895778}, "UV"={"u"=0.0, "v"=0.0}, "Colour"=12517256}, "Vertex 3"={"Position"={"x"=189.80782, "y"=199.68152, "z"=0.98959744}, "UV"={"u"=0.0, "v"=0.0}, "Colour"=12517256}, "Alpha"=0.0, "Alpha Blending Enabled"=FALSE, "Colour"=6456390}, {"Vertex 1"={"Position"={"x"=187.80107, "y"=204.32404, "z"=0.9895778}, "UV"={"u"=0.0, "v"=0.0}, "Colour"=12517256}, "Vertex 2"={"Position"={"x"=168.53177, "y"=213.96883, "z"=0.9895778}, "UV"={"u"=0.0, "v"=0.0}, "Colour"=12517256}, "Vertex 3"={"Position"={"x"=168.51642, "y"=218.47636, "z"=0.98959744}, "UV"={"u"=0.0, "v"=0.0}, "Colour"=12517256}, "Alpha"=0.0, "Alpha Blending Enabled"=FALSE, "Colour"=10606707}, {"Vertex 1"={"Position"={"x"=151.49875, "y"=224.43393, "z"=0.9895778}, "UV"={"u"=0.0, "v"=0.0}, "Colour"=12517256}, "Vertex 2"={"Position"={"x"=168.53177, "y"=213.96883, "z"=0.9895778}, "UV"={"u"=0.0, "v"=0.0}, "Colour"=12517256}, "Vertex 3"={"Position"={"x"=169.41815, "y"=209.785, "z"=0.98959744}, "UV"={"u"=0.0, "v"=0.0}, "Colour"=12517256}, "Alpha"=0.0, "Alpha Blending Enabled"=FALSE, "Colour"=6456390}, {"Vertex 1"={"Position"={"x"=168.53177, "y"=213.96883, "z"=0.9895778}, "UV"={"u"=0.0, "v"=0.0}, "Colour"=12517256}, "Vertex 2"={"Position"={"x"=151.49875, "y"=224.43393, "z"=0.9895778}, "UV"={"u"=0.0, "v"=0.0}, "Colour"=12517256}, "Vertex 3"={"Position"={"x"=152.57072, "y"=228.54994, "z"=0.98959744}, "UV"={"u"=0.0, "v"=0.0}, "Colour"=12517256}, "Alpha"=0.0, "Alpha Blending Enabled"=FALSE, "Colour"=10475122}, {"Vertex 1"={"Position"={"x"=136.65297, "y"=235.5601, "z"=0.9895778}, "UV"={"u"=0.0, "v"=0.0}, "Colour"=12517256}, "Vertex 2"={"Position"={"x"=151.49875, "y"=224.43393, "z"=0.9895778}, "UV"={"u"=0.0, "v"=0.0}, "Colour"=12517256}, "Vertex 3"={"Position"={"x"=151.36185, "y"=220.60233, "z"=0.98959744}, "UV"={"u"=0.0, "v"=0.0}, "Colour"=12517256}, "Alpha"=0.0, "Alpha Blending Enabled"=FALSE, "Colour"=6653768}, {"Vertex 1"={"Position"={"x"=151.49875, "y"=224.43393, "z"=0.9895778}, "UV"={"u"=0.0, "v"=0.0}, "Colour"=12517256}, "Vertex 2"={"Position"={"x"=136.65297, "y"=235.5601, "z"=0.9895778}, "UV"={"u"=0.0, "v"=0.0}, "Colour"=12517256}, "Vertex 3"={"Position"={"x"=138.70209, "y"=239.3482, "z"=0.98959744}, "UV"={"u"=0.0, "v"=0.0}, "Colour"=12517256}, "Alpha"=0.0, "Alpha Blending Enabled"=FALSE, "Colour"=10343024}, {"Vertex 1"={"Position"={"x"=123.94555, "y"=247.18822, "z"=0.9895778}, "UV"={"u"=0.0, "v"=0.0}, "Colour"=12517256}, "Vertex 2"={"Position"={"x"=136.65297, "y"=235.5601, "z"=0.9895778}, "UV"={"u"=0.0, "v"=0.0}, "Colour"=12517256}, "Vertex 3"={"Position"={"x"=135.59482, "y"=232.01439, "z"=0.98959744}, "UV"={"u"=0.0, "v"=0.0}, "Colour"=12517256}, "Alpha"=0.0, "Alpha Blending Enabled"=FALSE, "Colour"=6917451}, {"Vertex 1"={"Position"={"x"=136.65297, "y"=235.5601, "z"=0.9895778}, "UV"={"u"=0.0, "v"=0.0}, "Colour"=12517256}, "Vertex 2"={"Position"={"x"=123.94555, "y"=247.18822, "z"=0.9895778}, "UV"={"u"=0.0, "v"=0.0}, "Colour"=12517256}, "Vertex 3"={"Position"={"x"=126.85683, "y"=250.67299, "z"=0.98959744}, "UV"={"u"=0.0, "v"=0.0}, "Colour"=12517256}, "Alpha"=0.0, "Alpha Blending Enabled"=FALSE, "Colour"=10145390}, {"Vertex 1"={"Position"={"x"=113.32741, "y"=259.15903, "z"=0.9895778}, "UV"={"u"=0.0, "v"=0.0}, "Colour"=12517256}, "Vertex 2"={"Position"={"x"=123.94555, "y"=247.18822, "z"=0.9895778}, "UV"={"u"=0.0, "v"=0.0}, "Colour"=12517256}, "Vertex 3"={"Position"={"x"=122.07298, "y"=243.90215, "z"=0.98959744}, "UV"={"u"=0.0, "v"=0.0}, "Colour"=12517256}, "Alpha"=0.0, "Alpha Blending Enabled"=FALSE, "Colour"=7246670}, {"Vertex 1"={"Position"={"x"=123.94555, "y"=247.18822, "z"=0.9895778}, "UV"={"u"=0.0, "v"=0.0}, "Colour"=12517256}, "Vertex 2"={"Position"={"x"=113.32741, "y"=259.15903, "z"=0.9895778}, "UV"={"u"=0.0, "v"=0.0}, "Colour"=12517256}, "Vertex 3"={"Position"={"x"=116.981316, "y"=262.32532, "z"=0.98959744}, "UV"={"u"=0.0, "v"=0.0}, "Colour"=12517256}, "Alpha"=0.0, "Alpha Blending Enabled"=FALSE, "Colour"=9947756}, {"Vertex 1"={"Position"={"x"=104.74968, "y"=271.31357, "z"=0.9895778}, "UV"={"u"=0.0, "v"=0.0}, "Colour"=12517256}, "Vertex 2"={"Position"={"x"=113.32741, "y"=259.15903, "z"=0.9895778}, "UV"={"u"=0.0, "v"=0.0}, "Colour"=12517256}, "Vertex 3"={"Position"={"x"=110.75225, "y"=256.14658, "z"=0.98959744}, "UV"={"u"=0.0, "v"=0.0}, "Colour"=12517256}, "Alpha"=0.0, "Alpha Blending Enabled"=FALSE, "Colour"=7510354}, {"Vertex 1"={"Position"={"x"=113.32741, "y"=259.15903, "z"=0.9895778}, "UV"={"u"=0.0, "v"=0.0}, "Colour"=12517256}, "Vertex 2"={"Position"={"x"=104.74968, "y"=271.31357, "z"=0.9895778}, "UV"={"u"=0.0, 
